vi "NameMap-Merge.vi"(6 "If exist? Skip(T)/Overwrite(F)":bool=TRUE, 8 "error in (no error)":errorcluster, 10 "NameMap B":T1, 11 "NameMap A":T1) -> (0 "error out":errorcluster, 3 "NameMap A after B->A":T1)   [LabVIEW 2019, in "lv-apt-json-file.lvlib"]
uses:
  lv-apt-json-file.lvlib
  Typedef/Def-NameMap.ctl
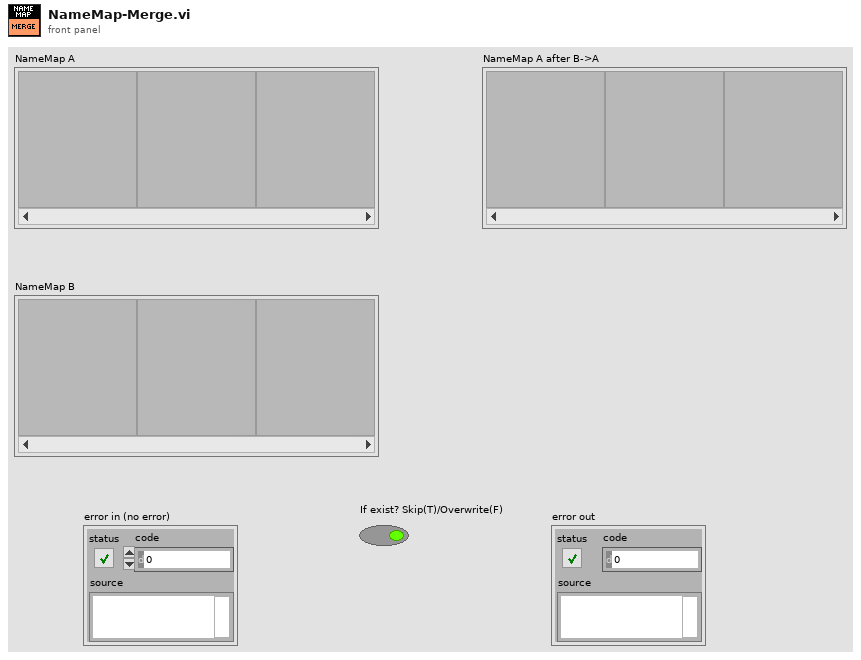
[diagram p1: front panel]
types:
  T1 = typedef "lv-apt-json-file.lvlib/Def-NameMap.ctl" = variant[]
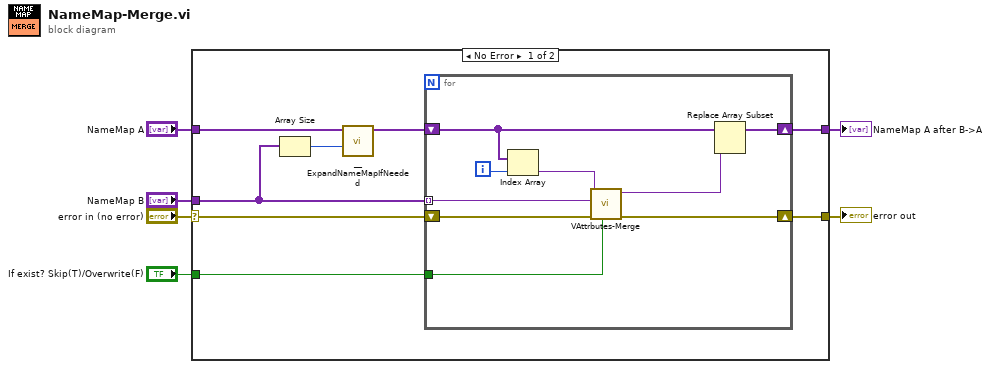
[diagram p0: block diagram]
diagram:
  n1 = case shown="No Error" "error in (no error)" {
    selector: "error in (no error)" -> [w7 w25]
    tunnel: "NameMap A" -> [w11 w24]
    tunnel: "NameMap B" -> [w13 _]
    tunnel: "If exist? Skip(T)/Overwrite(F)" -> [w14 _]
    tunnel: [w8 w25] -> w2
    tunnel: [w9 w24] -> w1
    frame No Error {
      n2 = Array Size(array=w13) -> (size(s)=w10:i32)
      n3 = call "__ExpandNameMapIfNeeded.vi"("Numeric"=w10, "NameMap A in"=w11) -> ("NameMap A out"=w12:T1)  [unwired: 9 in]
      n4 = for {
        tunnel: w14 -> [w17]
        shift-right: [w19] -> w9
        shift-left: w12 -> [w22]
        tunnel: w13 -> [w23] mode=indexing
        shift-right: [w16] -> w8
        shift-left: w7 -> [w15]
        i -> [w21]
        n5 = Index Array(array=w22, index=w21) -> (element=w20:variant)
        n6 = call "VAttrbutes-Merge.vi"("If exist? Skip(T)/Overwrite(F)"=w17, "error in (no error)"=w15, "VAttributes B"=w23, "VAttributes A"=w20) -> ("error out"=w16:errorcluster, "VAttributes A after B->A"=w18:variant)  [unwired: 6 in]
        n7 = Replace Array Subset(array=w22, new element=w18) -> (w19:T1)  [unwired: 1 in]
      }
    }
    frame Error {
    }
  }
  "NameMap A after B->A" <- w1
  "error out" <- w2
